vi "T257P_Set_Chiller_Status.vi"(0 "T257P Port IN":refnum<visa-resource-name>, 1 "Chiller Status":bool, 5 "error in (no error)":errorcluster) -> (7 "Sent buffer 1":string, 11 "Read buffer 1":string, 14 "T257P Port OUT":refnum<visa-resource-name>, 15 "Chiller Status":bool, 16 "CheckSum 1":string, 19 "error out":errorcluster)   [LabVIEW 2020]
doc: "ThermoTek T257P Labview Driver Library. © G.Shtengel. gleb.shtengel@gmail.com"
panel:
  out "Loop Counter 1":i32
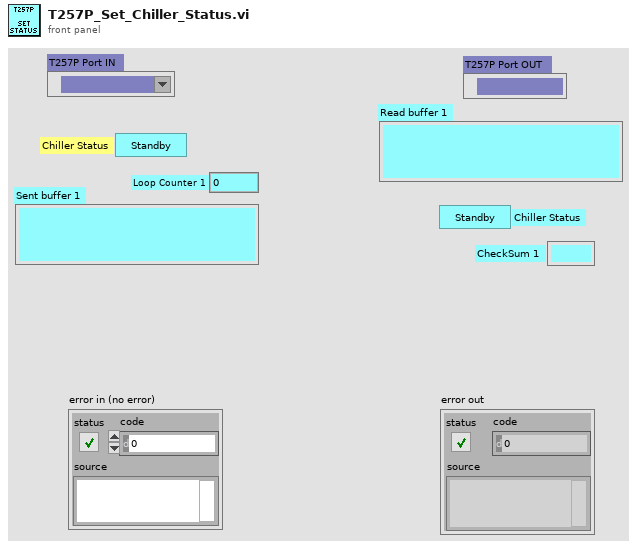
[diagram p1: front panel]
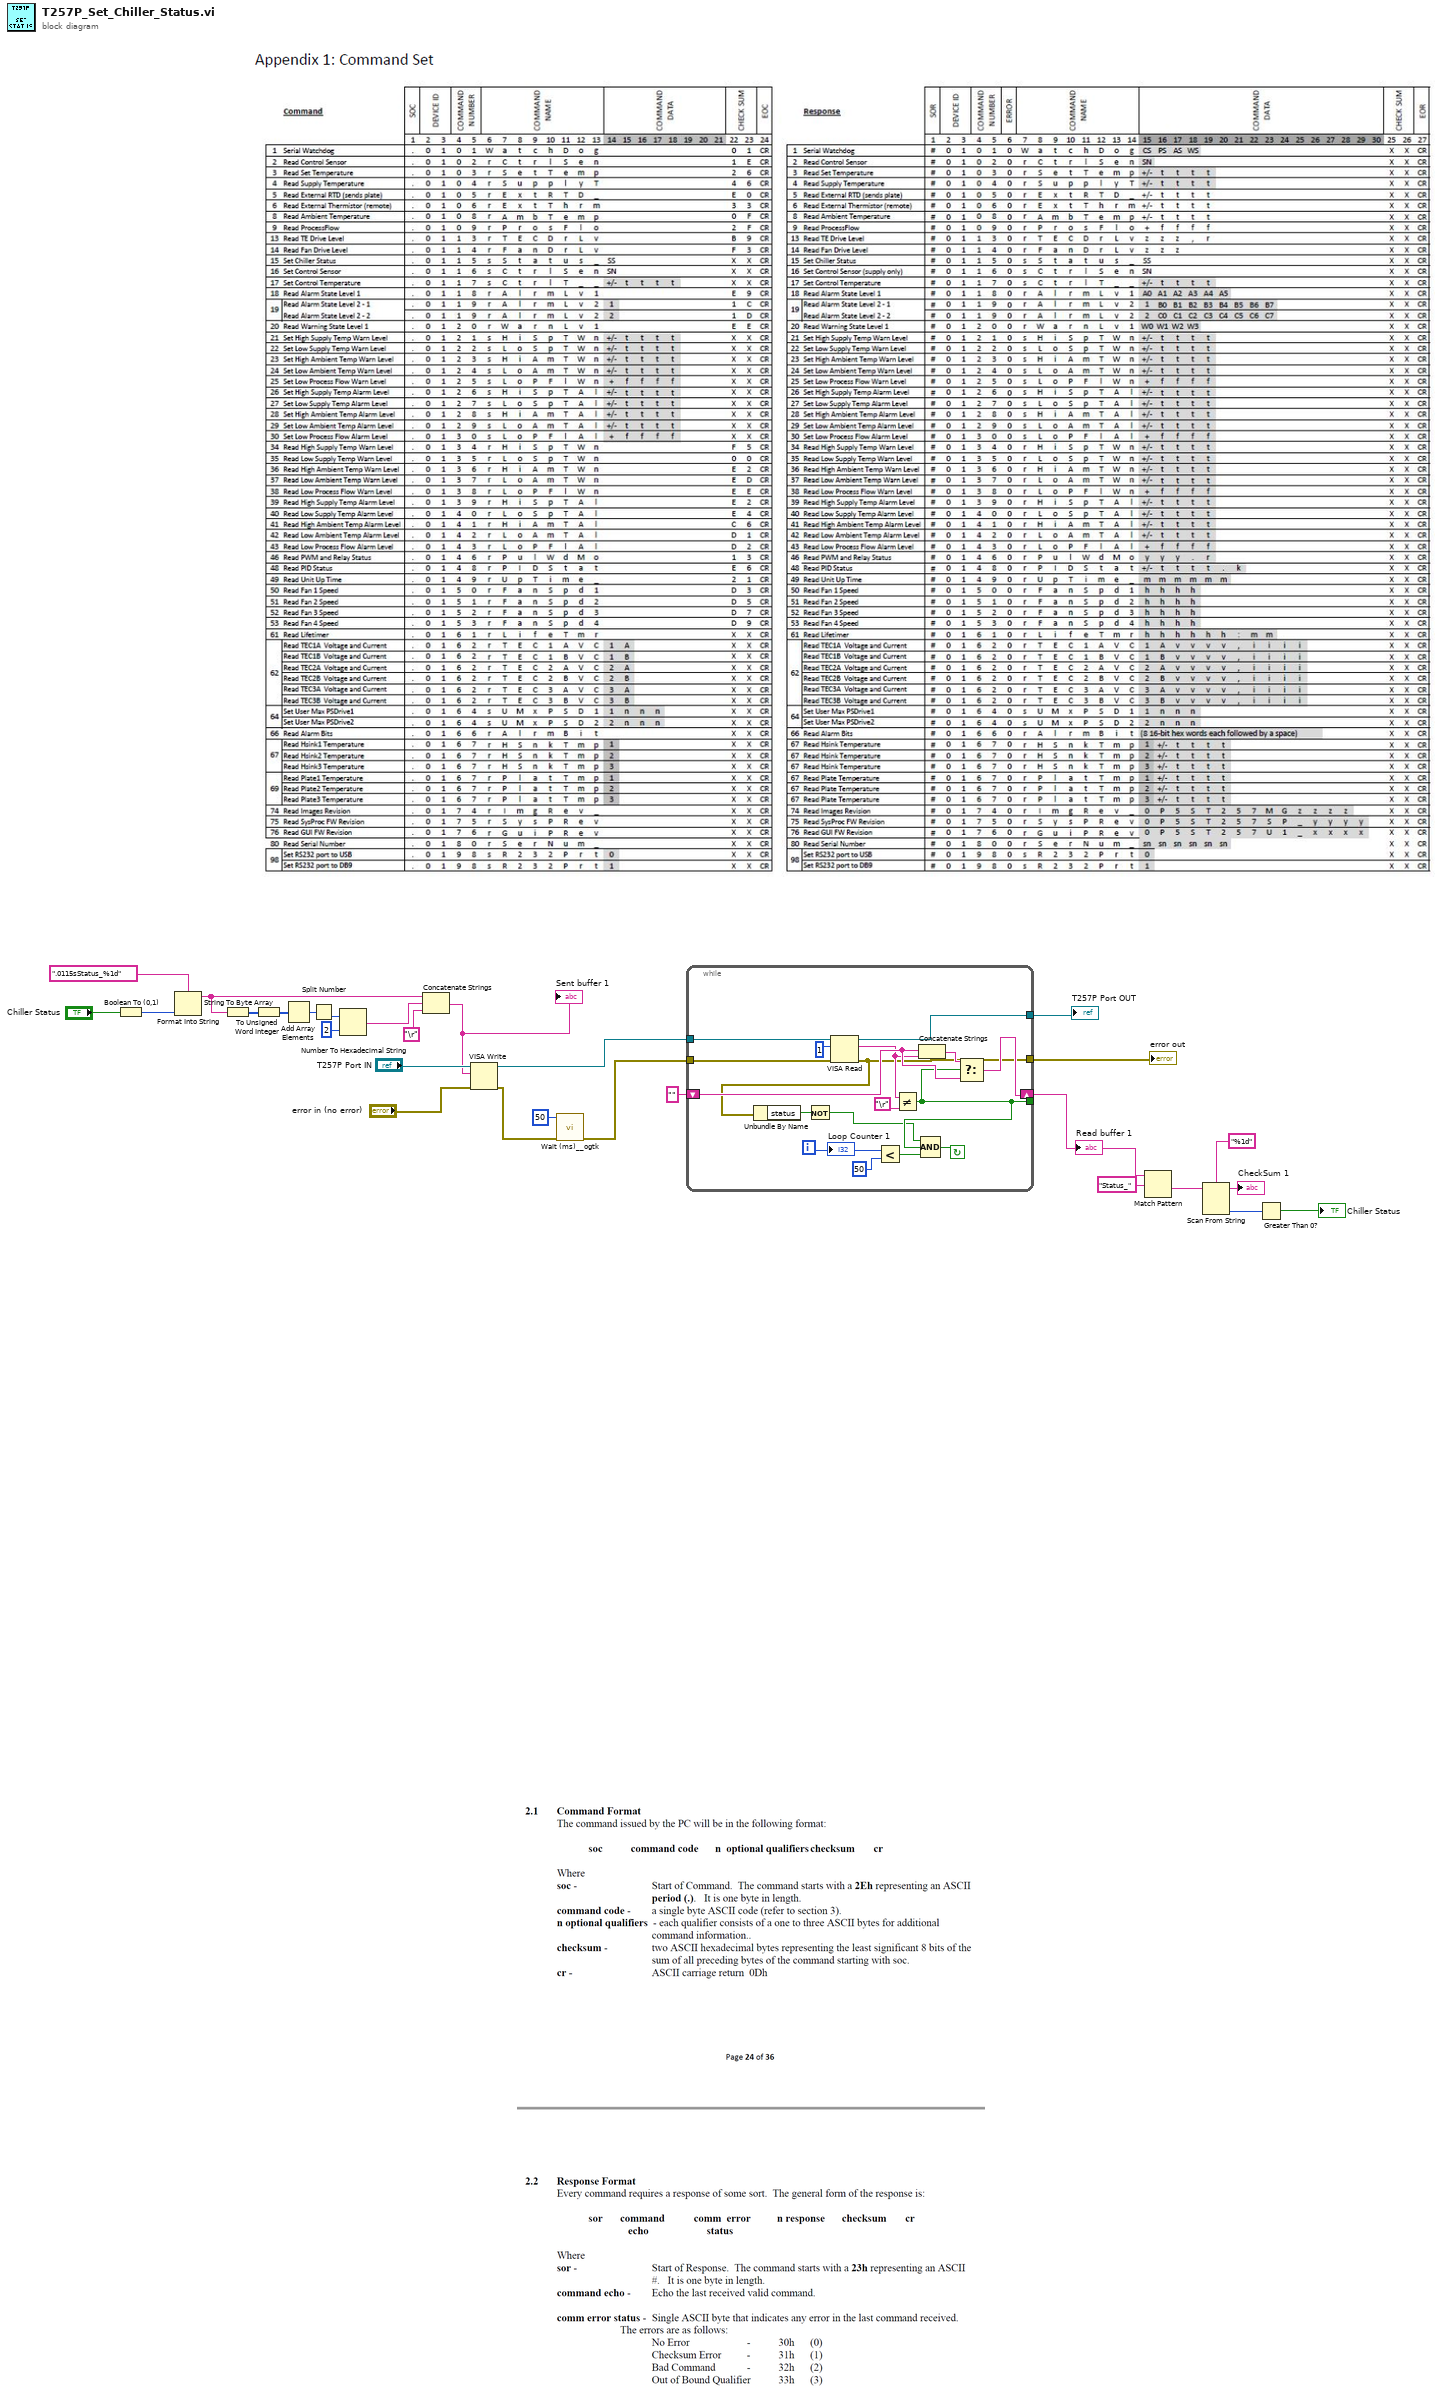
[diagram p0: block diagram]
diagram:
  n1 = Boolean To (0,1)(Boolean="Chiller Status") -> (0, 1=w2:i16)
  n2 = Format Into String(format string=".0115sStatus_%1d" ("Sent buffer 2"), w2) -> (resulting string=w10:string)  [unwired: 2 in, 1 out]
  n3 = String To Byte Array(string=w10) -> (unsigned byte array=w14:u8[])
  n4 = To Unsigned Word Integer(number=w14) -> (unsigned 16bit integer=w13:u16[])
  n5 = Add Array Elements(numeric array=w13) -> (sum=w12:u16)
  n6 = Split Number(x=w12) -> (lo(x)=w11:u8)  [unwired: 1 out]
  n7 = Number To Hexadecimal String(1:i16 2 ("width (-)"), 2:w11) -> (0:w9:string)
  n8 = Concatenate Strings(w10, w9, "\r") -> (w7:string)
  "Sent buffer 1" <- w7
  n9 = VISA Write(VISA resource name="T257P Port IN", write buffer=w7, error in (no error)="error in (no error)") -> (VISA resource name out=w24:refnum<visa-resource-name>, error out=w25:errorcluster)  [unwired: 1 out]
  n10 = call <userlib>:"Wait (ms)__ogtk.vi"("error in (no error)"=w25, "milliseconds to wait"=u32 50) -> ("error out"=w23:errorcluster)  [unwired: 8 in, 1 out]
  n11 = while {
    shift-left: "" -> [w42]
    shift-right: [w41] -> w18
    tunnel: [w39] -> _
    tunnel: [w31] -> w15
    tunnel: [w40] -> w16
    tunnel: w24 -> [w37]
    tunnel: w23 -> [w36]
    i -> [w38]
    stop <- w43 continue-if-true
    n12 = VISA Read(VISA resource name=w37, byte count=u32 1 ("byte count (0)"), error in (no error)=w36) -> (VISA resource name out=w40:refnum<visa-resource-name>, read buffer=w34:string, error out=w31:errorcluster)  [unwired: 1 out]
    n13 = Unbundle By Name(w31) -> ("status"=w30:bool)
    n14 = Not(x=w30) -> (.not. x?=w29:bool)
    n15 = Less?(x=w38, y=50) -> (x < y?=w44:bool)
    n16 = Not Equal?(x=w34, y="\r") -> (x != y?=w39:bool)
    n17 = Concatenate Strings(w42, w34) -> (w32:string)
    n18 = Compound Arithmetic op=AND(w29, w39, w44) -> (w43:bool)
    n19 = Select(t=w32, s=w39, f=w42) -> (s? t:f=w41:string)
    "Loop Counter 1" <- w38
  }
  "error out" <- w15
  "Read buffer 1" <- w18
  "T257P Port OUT" <- w16
  n20 = Match Pattern(string=w18, regular expression="Status_") -> (after substring=w19:string)  [unwired: 1 in, 3 out]
  n21 = Scan From String(format string="%1d", input string=w19) -> (remaining string=→"CheckSum 1":string, output 1=w3:i32)  [unwired: 3 in, 2 out]
  n22 = Greater Than 0?(x=w3) -> (x > 0?=→"Chiller Status":bool)
